vi "Register ATML DataPlugin.vi"(8 "error in":errorcluster, 11 "path":path) -> (0 "error out":errorcluster)   [LabVIEW 2023]
doc: "When run as an executable, this VI takes command line arguments and passes them to the Register DataPlugin VI to register a new DataPlugin on the computer running the executable. When run as a VI, it registers the DataPlugin specified by path."
uses:
  <vilib>/Platform/storage/utility/Register DataPlugin by URI.vi
panel:
  # "When running this VI as part of the Read ATML File.vi example, drag the Support Files > ATML_5.uri project item from DataPlugins - ATML.lvproj into the path control below and run this VI. Then, follow the remaining instructions on the front panel of Read ATML File.vi."
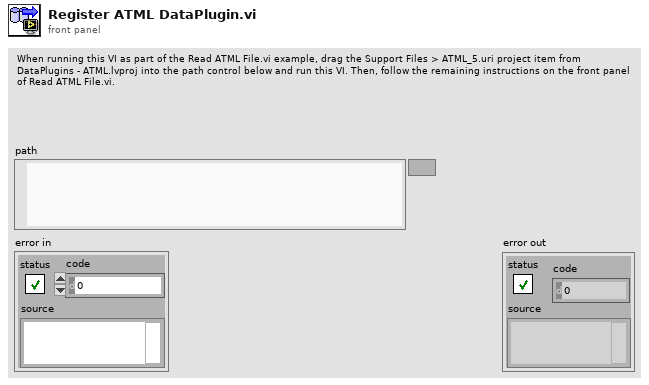
[diagram p1: front panel]
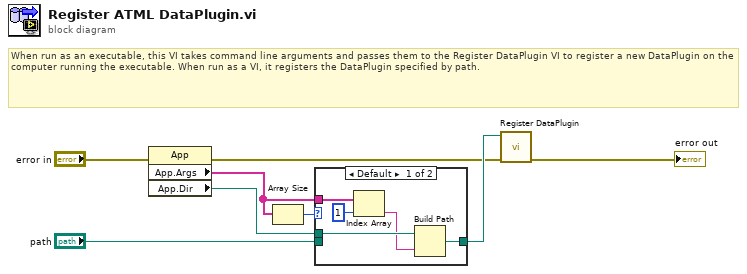
[diagram p0: block diagram]
diagram:
  # "When run as an executable, this VI takes command line arguments and passes them to the Register DataPlugin VI to register a new DataPlugin on the computer running the executable. When run as a VI, it registers the DataPlugin specified by path."
  n1 = property class="App"(error in="error in") -> (error out=w1:errorcluster, "App.Args"=w5:string[], "App.Dir"=w4:path)  [unwired: 1 in, 1 out]
  n2 = Array Size(array=w5) -> (size(s)=w8:i32)
  n3 = case shown="Default" w8 {
    tunnel: "path" -> [_ w14]
    tunnel: [w9 w14] -> w6
    tunnel: w5 -> [w13 _]
    tunnel: w4 -> [w11 _]
    frame Default {
      n4 = Index Array(array=w13, index=1) -> (element=w10:string)
      n5 = Build Path(base path=w11, name or relative path=w10) -> (appended path=w9:path)
    }
    frame 1 {
    }
  }
  n6 = call-poly <vilib>:"Register DataPlugin.vi"("error in (no error)"=w1, "DataPlugin URI path (*.uri)"=w6) -> ("error out"=→"error out":errorcluster)  [unwired: 7 in, 2 out]
